vi "NumToRefnum.vi"(1 "Reference ID":u64) -> (0 "Refnum Out":refnum<k20>)   [LabVIEW 2023]
doc: "Converts numeric reference ID to FPGA refnum"
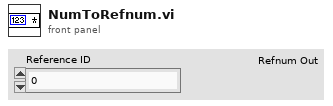
[diagram p1: front panel]
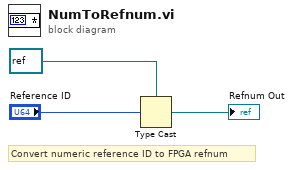
[diagram p0: block diagram]
diagram:
  # "Convert numeric reference ID to FPGA refnum"
  n1 = Type Cast(type=refnum<k20> refnum ("Refnum in"), x="Reference ID") -> (*(type *) &x=→"Refnum Out":refnum<k20>)
